vi "Kinect Find Contours.vi"(0 "Image Src":T1, 5 "Height Threshold":dbl(slide) min=-32768.0 max=32768.0 step=1.0 scale=0.0..300.0, 7 "Contour Length Threshold":dbl(slide) min=-32768.0 max=32768.0 step=1.0 scale=0.0..500.0, 9 "Width":u32=1, 11 "error in (no error)":errorcluster) -> (4 "Image Out":T1, 6 "Curves":T2[](array[typedef]) {"Points"."Y" format="%.2f"; "Points"."X" format="%.2f"}, 15 "error out":errorcluster)   [LabVIEW 2011]
uses:
  <vilib>/vision/Analysis.llb/IMAQ ExtractCurvesCurve.ctl
  <vilib>/vision/Image Controls.llb/IMAQ Image.ctl
  <vilib>/vision/Pattern Matching.llb/IMAQ Curve Parameters.ctl
  <vilib>/vision/NI_Vision_Development_Module.lvlib
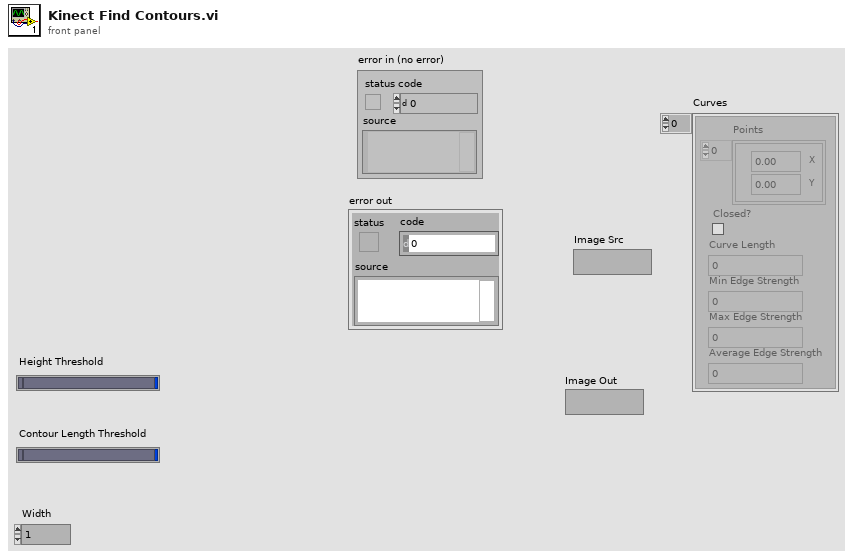
[diagram p1: front panel]
types:
  T1 = typedef "IMAQ Image.ctl" = refnum<image>
  T2 = typedef "IMAQ ExtractCurvesCurve.ctl" = cluster{"Points":cluster{"X":dbl, "Y":dbl}[], "Closed?":bool, "Curve Length":dbl, "Min Edge Strength":dbl, "Max Edge Strength":dbl, "Average Edge Strength":dbl}
  T3 = typedef "Image Type" = u32
  T4 = typedef "IMAQ Curve Parameters.ctl" = cluster{"Extraction Mode":u32, "Edge Threshold":i32, "Edge Filter Size":u32, "Min Length":i32, "Row Search Step Size":i32, "Col Search Step Size":i32, "Max Endpoint Gap":i32, "Closed":bool, "Subpixel":bool}
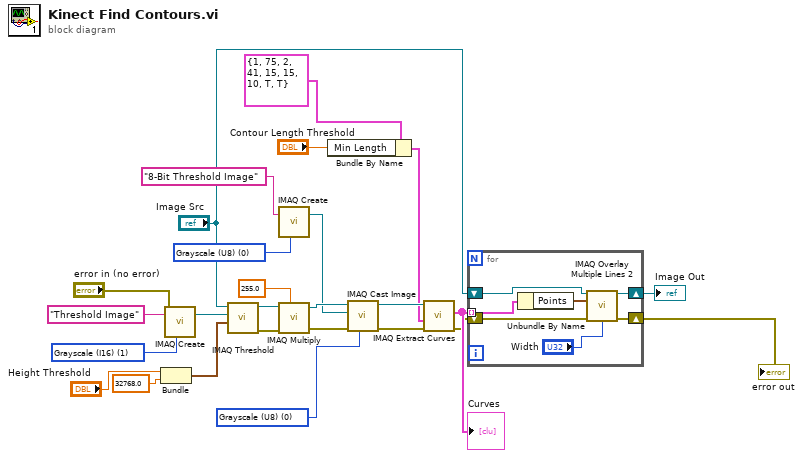
[diagram p0: block diagram]
diagram:
  w7 = T3 0 items=["Grayscale (U8)", "Grayscale (I16)", "Grayscale (SGL)", "Complex (CSG)", "RGB (U32)", "HSL (U32)", "RGB (U64)", "Grayscale (U16)"] ("Image Type")
  w10 = T3 1 items=["Grayscale (U8)", "Grayscale (I16)", "Grayscale (SGL)", "Complex (CSG)", "RGB (U32)", "HSL (U32)", "RGB (U64)", "Grayscale (U16)"] ("Image Type")
  w21 = T3 0 items=["Grayscale (U8)", "Grayscale (I16)", "Grayscale (SGL)", "Complex (CSG)", "RGB (U32)", "HSL (U32)", "RGB (U64)", "Grayscale (U16)"] ("Image Type")
  n1 = Bundle("Height Threshold"="Height Threshold", "element"=32768.0) -> (w24:cluster{"Height Threshold":dbl, "element":dbl})  [unwired: 1 in]
  n2 = call "IMAQ Create"("Image Name"="Threshold Image", "Image Type"=w10, "error in (no error)"="error in (no error)") -> ("New Image"=w8:T1)  [unwired: 2 in, 1 out]
  n3 = call "IMAQ Threshold"("Range"=w24, "Image Dst"=w8, "Image Src"="Image Src") -> ("error out"=w16:errorcluster, "Image Dst Out"=w19:T1)  [unwired: 7 in]
  n4 = call "IMAQ Create"("Image Name"="8-Bit Threshold Image", "Image Type"=w7) -> ("New Image"=w5:T1)  [unwired: 3 in, 1 out]
  n5 = call "IMAQ Multiply"("Image Src A"=w19, "Constant"=sgl 255.0, "error in (no error)"=w16) -> ("Image Dst Out"=w18:T1, "error out"=w17:errorcluster)  [unwired: 4 in]
  n6 = Bundle By Name(cluster=T4 {"Extraction Mode"=1, "Edge Threshold"=75, "Edge Filter Size"=2, "Min Length"=41, "Row Search Step Size"=15, "Col Search Step Size"=15, "Max Endpoint Gap"=10, "Closed"=TRUE, "Subpixel"=TRUE} ("Curve Parameters"), "Min Length"="Contour Length Threshold") -> (w14:T4)
  n7 = call "IMAQ Cast Image"("Image Type"=w21, "error in (no error)"=w17, "Image Dst"=w5, "Image Src"=w18) -> ("error out"=w23:errorcluster, "Image Dst Out"=w26:T1)  [unwired: 6 in]
  n8 = call "IMAQ Extract Curves"("error in (no error)"=w23, "Curve Parameters"=w14, "Image"=w26) -> ("error out"=w2:errorcluster, "Curves"=w22:T2[])  [unwired: 6 in, 1 out]
  "Curves" <- w22
  n9 = for {
    shift-right: [w30] -> w4
    shift-left: "Image Src" -> [w32]
    tunnel: w22 -> [w29] mode=indexing
    shift-right: [w27] -> w1
    shift-left: w2 -> [w28]
    n10 = Unbundle By Name(w29) -> ("Points"=w33:cluster{"X":dbl, "Y":dbl}[])
    n11 = call "IMAQ Overlay Multiple Lines 2"("Image"=w32, "Line End Points"=w33, "error in (no error)"=w28, "Width"="Width") -> ("Image Out"=w30:T1, "error out"=w27:errorcluster)  [unwired: 10 in]
  }
  "Image Out" <- w4
  "error out" <- w1
